vi "Actor Core.vi"(8 "error in":errorcluster, 11 "Keithley Meter in":refnum<class "Keithley Meter.lvclass">) -> (0 "error out":errorcluster, 3 "Actor out":refnum<class "Actor.lvclass">)   [LabVIEW 2015, in "Keithley Meter.lvclass"]
doc: "(<B>Filename</B>: Actor Framework.lvlib:Actor.lvclass:Actor Core.vi)\n\nReceives messages to the actor, reacts to them, and initiates any error handling that may shut the actor down.\n\nDescendant classes may override this VI to append parallel tasks for the actor to complete while it handles messages. Overrides use the Call Parent Method node."
uses:
  Keithley Meter.lvclass
  <vilib>/ActorFramework/Actor/Actor.lvclass
  NHMFL_Core/Libraries/Instruments/Keithley/Meter/Keithley Meter Parameters.ctl
  NHMFL_Core/Libraries/Instruments/Keithley/Meter/KeithleyMeter Function.ctl
  Meter/Meter.lvclass
panel:
  in  "Parameters":T1={"Range (-1: auto)"=-1.0, "Integration Time (NPLCs)"=1.0, "Function"=enum."VOLTAGE", "W Offset comp"=FALSE, "4-wire W"=FALSE, "Scale"=1.0, "Offset"=0.0} {"Integration Time (NPLCs)" min=0.01 max=10.0 step=0.01 format="%.2f"}
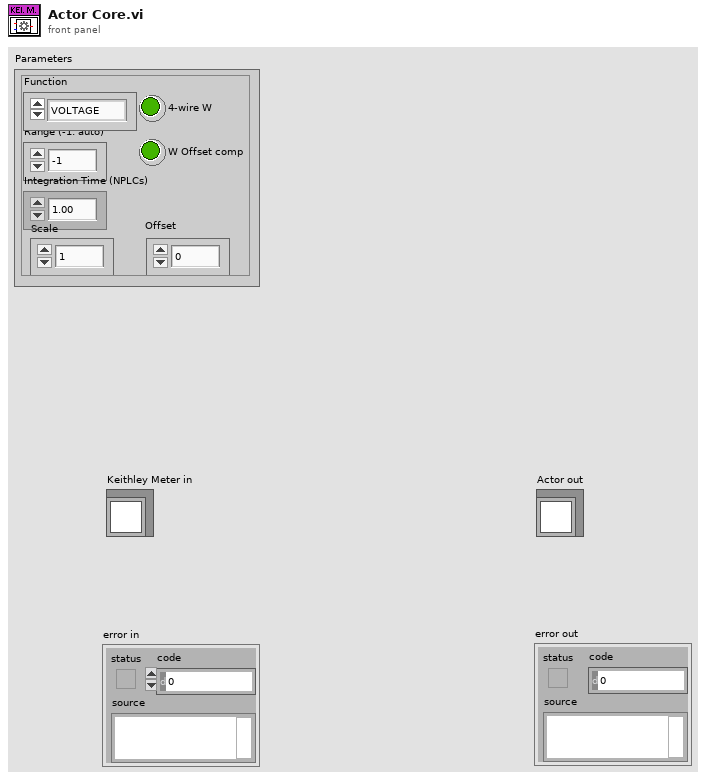
[diagram p1: front panel]
types:
  T1 = typedef "Keithley Meter Parameters.ctl" = cluster{"Range (-1: auto)":dbl, "Integration Time (NPLCs)":dbl, "Function":T2, "W Offset comp":bool, "4-wire W":bool, "Scale":dbl, "Offset":dbl}
  T2 = typedef "KeithleyMeter Function.ctl" = enum16{"VOLTAGE", "CURRENT", "RESISTANCE"}
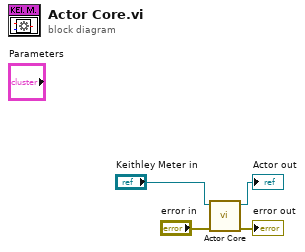
[diagram p0: block diagram]
diagram:
  n1 = call-parent "Actor Core.vi"("error in"="error in", "Meter in"="Keithley Meter in") -> ("error out"=→"error out":errorcluster, "Actor out"=→"Actor out":refnum<class "Actor.lvclass">)  [unwired: 8 in]
